vi "add_data.vi"(7 "n_max":i32, 8 "value":dbl, 9 "timestamp":timestamp, 11 "array_in":T1(array[cluster])) -> (0 "cluster_out":cluster{"timestamp":timestamp, "value":dbl}, 3 "array_out":T1(array[cluster]))   [LabVIEW 2019]
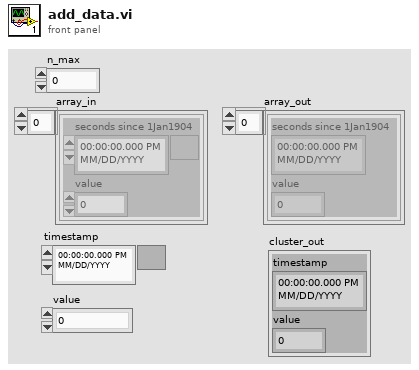
[diagram p1: front panel]
types:
  T1 = cluster{"seconds since 1Jan1904":timestamp, "value":dbl}[]
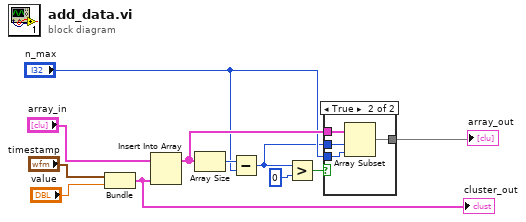
[diagram p0: block diagram]
diagram:
  n1 = Bundle("timestamp"="timestamp", "value"="value") -> (w11:cluster{"timestamp":timestamp, "value":dbl})  [unwired: 1 in]
  "cluster_out" <- w11
  n2 = Insert Into Array(array="array_in", new element=w11) -> (w6:T1)  [unwired: 1 in]
  n3 = Array Size(array=w6) -> (size(s)=w5:i32)
  n4 = Subtract(x=w5, y="n_max") -> (x-y=w3:i32)
  n5 = Greater?(x=w3, y=0) -> (0:w1:bool)
  n6 = case shown="True" w1 {
    tunnel: [w12 w16] -> w7
    tunnel: w6 -> [w12 w15]
    tunnel: "n_max" -> [_ w14]
    tunnel: w3 -> [_ w13]
    frame False {
    }
    frame True {
      n7 = Array Subset(array=w15, index=w13, length=w14) -> (w16:T1)
    }
  }
  "array_out" <- w7
